vi "Convert Bitpacked U32 DMA.vi"(10 "Channels":i32, 11 "binary array":u32[](array[numeric])) -> (3 "Data":u8[][](array[numeric]))   [LabVIEW 2015, in "FPGA Addon Engine.lvlib"]
uses:
  FPGA Addon Engine.lvlib
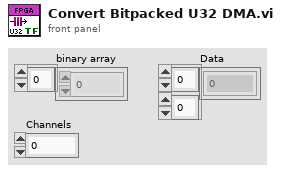
[diagram p1: front panel]
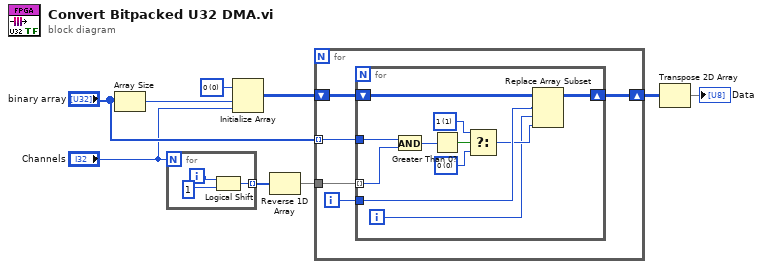
[diagram p0: block diagram]
diagram:
  w4 = u8 0 items=["0", "1", "Z", "L", "H", "X", "T", "V"] ("Digital Values")
  n1 = Array Size(array="binary array") -> (size(s)=w3:i32)
  n2 = for {
    N: "Channels" -> [_]
    tunnel: [w10] -> w1 mode=indexing
    i -> [w11]
    n3 = Logical Shift(y=w11, x=u32 1) -> (x << y=w10:u32)
  }
  n4 = Initialize Array(w4, w3, "Channels") -> (w5:u8[][])
  n5 = Reverse 1D Array(array=w1) -> (reversed array=w2:u32[])
  n6 = for {
    tunnel: "binary array" -> [w17] mode=indexing
    tunnel: w2 -> [w16]
    shift-right: [w13] -> w6
    shift-left: w5 -> [w15]
    i -> [w14]
    n7 = for {
      tunnel: w17 -> [w28]
      tunnel: w16 -> [w27] mode=indexing
      shift-right: [w19] -> w13
      shift-left: w15 -> [w22]
      tunnel: w14 -> [w21]
      i -> [w18]
      w24 = u8 0 items=["0", "1", "Z", "L", "H", "X", "T", "V"] ("Digital Values")
      w23 = u8 1 items=["0", "1", "Z", "L", "H", "X", "T", "V"] ("Digital Values")
      n8 = And(x=w28, y=w27) -> (x .and. y?=w26:u32)
      n9 = Greater Than 0?(x=w26) -> (x > 0?=w25:bool)
      n10 = Select(t=w23, s=w25, f=w24) -> (s? t:f=w20:u8)
      n11 = Replace Array Subset(array=w22, new element=w20, index (row)=w21, index (col)=w18) -> (w19:u8[][])
    }
  }
  n12 = Transpose 2D Array(2D array=w6) -> (transposed array=→"Data":u8[][])
